vi "UTILITY Fuzzy Logic Scale.vi"(7 "Convert to MicroAmp (T), Standard Output (F)":bool, 8 "Error In":errorcluster, 10 "input variable":dbl, 11 "output range":cluster{"output high":dbl, "output low":dbl}={"output high"=140.0, "output low"=40.0} {"output low" format="%.2f"; "output high" format="%.2f"}) -> (0 "Error Out":errorcluster, 3 "MicroAmp":dbl)   [LabVIEW 2018]
uses:
  <vilib>/Analysis/NI_AALPro.lvlib
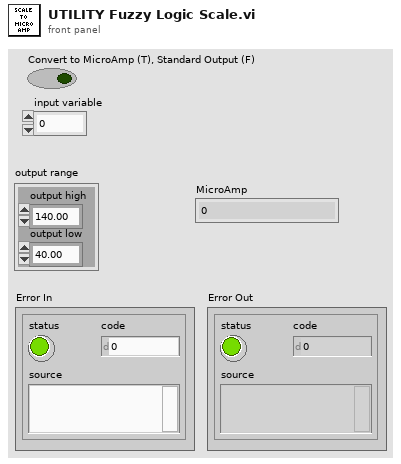
[diagram p1: front panel]
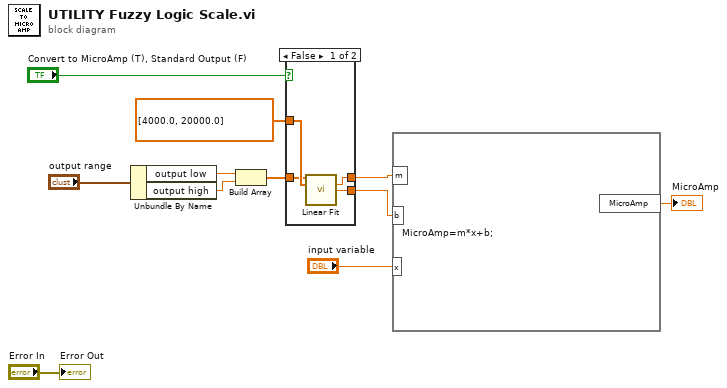
[diagram p0: block diagram]
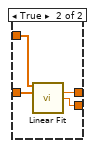
[diagram p2: hidden frame]
diagram:
  n1 = Unbundle By Name("output range") -> ("output low"=w5:dbl, "output high"=w4:dbl)
  n2 = Build Array(w5, w4) -> (w3:dbl[])
  n3 = case shown="False" "Convert to MicroAmp (T), Standard Output (F)" {
    tunnel: dbl[] [4000.0, 20000.0] ("Y") -> [w15 w19]
    tunnel: [w13 w18] -> w9
    tunnel: [w12 w17] -> w8
    tunnel: w3 -> [w14 w16]
    frame False {
      n4 = call <vilib>:"Linear Fit.vi"("Y"=w14, "X"=w15) -> ("slope"=w13:dbl, "intercept"=w12:dbl)  [unwired: 9 in, 3 out]
    }
    frame True {
      n5 = call <vilib>:"Linear Fit.vi"("Y"=w19, "X"=w16) -> ("slope"=w18:dbl, "intercept"=w17:dbl)  [unwired: 9 in, 3 out]
    }
  }
  n6 = formula code="MicroAmp=m*x+b;"("m"=w9, "b"=w8, "x"="input variable") -> ("MicroAmp"=→"MicroAmp":dbl)
  "Error Out" <- "Error In"
